vi "Draw ROIs.vi"(8 "error in (no error)":errorcluster, 9 "Numeric":i32, 10 "index of element":i32, 11 "Refnum in":T1) -> (0 "error out":errorcluster, 2 "ROI Descriptor":T2 {"Contours"."Type" items=["No Selection", "Point", "Line", "Rectangle", "Oval", "Polygon", "Freehand Region", "Annulus", "Unused2", "Unused3", "Broken Line", "Freehand Line", "Rotated Rectangle"]}, 3 "Refnum out":T1)   [LabVIEW 2018, in "Image Management.lvlib"]
uses:
  Image Management.lvlib
  <vilib>/vision/Image Controls.llb/IMAQ Image.ctl
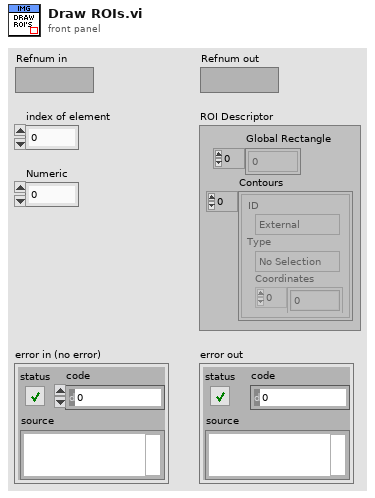
[diagram p1: front panel]
types:
  T1 = typedef "IMAQ Image.ctl" = refnum<image>
  T2 = typedef "ROI Descriptor" = cluster{"Global Rectangle":i32[], "Contours":cluster{"ID":enum32{"External", "Internal"}, "Type":u32, "Coordinates":i32[]}[]}
  T3 = typedef "IMAQ Rectangle" = cluster{"Left":i32, "Top":i32, "Right":i32, "Bottom":i32, "Rotation":dbl}
  T4 = cluster{"Left":i32, "Top":i32, "Right":i32, "Bottom":i32}
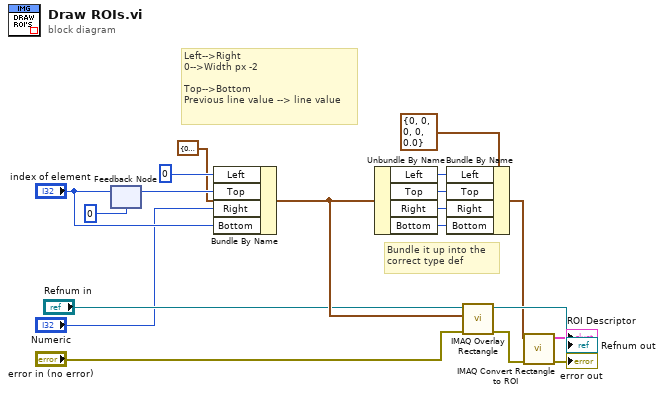
[diagram p0: block diagram]
diagram:
  # "Bundle it up into the \ncorrect type def"
  # "Left-->Right\n0-->Width px -2\n\nTop-->Bottom\nPrevious line value --> line value"
  n1 = feedback #1(0 ("index of element")) -> (w4:i32)
  n2 = feedback-in #1("index of element") -> ()
  n3 = Bundle By Name(cluster=T4 {"Left"=0, "Top"=0, "Right"=0, "Bottom"=0} ("Rectangle"), "Left"=0 ("element"), "Top"=w4, "Right"="Numeric", "Bottom"="index of element") -> (w9:T4)
  n4 = Unbundle By Name(w9) -> ("Left"=w11:i32, "Top"=w12:i32, "Right"=w13:i32, "Bottom"=w14:i32)
  n5 = Bundle By Name(cluster=T3 {"Left"=0, "Top"=0, "Right"=0, "Bottom"=0, "Rotation"=0.0} ("Rectangle"), "Left"=w11, "Top"=w12, "Right"=w13, "Bottom"=w14) -> (w10:T3)
  n6 = call "IMAQ Overlay Rectangle"("error in (no error)"="error in (no error)", "Rectangle"=w9, "Image"="Refnum in") -> ("error out"=w15:errorcluster, "Image Out"=→"Refnum out":T1)  [unwired: 7 in]
  n7 = call "IMAQ Convert Rectangle to ROI"("error in (no error)"=w15, "Rectangle"=w10) -> ("error out"=→"error out":errorcluster, "ROI Descriptor"=→"ROI Descriptor":T2)  [unwired: 7 in]
